vi "Position Fly Button Underneath.vi"(8 "error in (no error)":errorcluster, 10 "Previous Button":refnum<vi>, 11 "Fly Button Ref":refnum<vi>) -> (0 "error out":errorcluster)   [LabVIEW 2014]
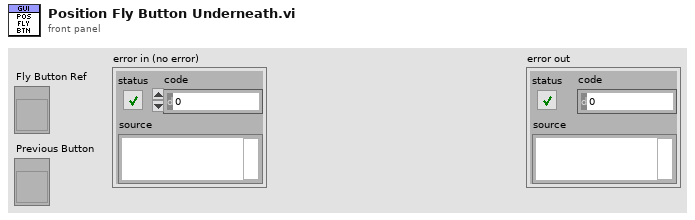
[diagram p1: front panel]
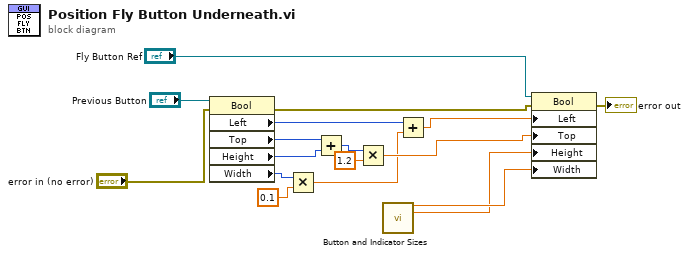
[diagram p0: block diagram]
diagram:
  n1 = property class="Bool"(reference="Previous Button", error in="error in (no error)") -> (error out=w16:errorcluster, "Left"=w5:i32, "Top"=w13:i32, "Height"=w11:u32, "Width"=w4:u32)  [unwired: 1 out]
  n2 = Multiply(x=w4, y=0.1) -> (x*y=w2:dbl)
  n3 = Add(x=w13, y=w11) -> (x+y=w8:u32)
  n4 = Multiply(x=w8, y=1.2) -> (x*y=w6:dbl)
  n5 = call "Button and Indicator Sizes.vi"() -> ("Button Width"=w10:dbl, "Button Height"=w9:dbl)  [unwired: 11 in, 3 out]
  n6 = Add(x=w5, y=w2) -> (x+y=w1:dbl)
  n7 = property class="Bool"(reference="Fly Button Ref", error in=w16, "Left"=w1, "Top"=w6, "Height"=w9, "Width"=w10) -> (error out=→"error out":errorcluster)  [unwired: 1 out]
